vi "单个流程写入.vi"(8 "error in (no error)":errorcluster, 10 "添加的路径":path, 11 "参数簇":T1={"启动参数"=1, "启动模式"=enum."跨度核查", "量程"=enum."低量程"} {"启动参数" items=["总磷"=1, "总氮"=2, "氨氮"=3]}) -> (0 "error out":errorcluster, 3 "步数":i32)   [LabVIEW 2016, in "斯坦道氨氮V2.lvlib"]
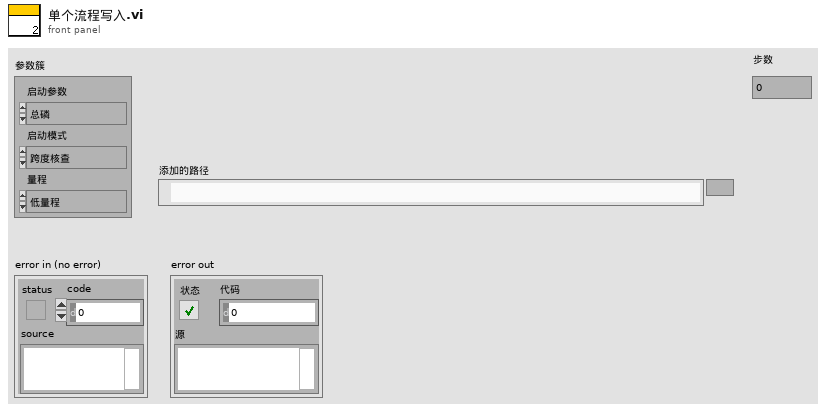
[diagram p1: front panel]
types:
  T1 = cluster{"启动参数":u16, "启动模式":enum16{"跨度核查", "水样测量", "零点核查", "标样核查", "加标回收", "快捷测试", "空白校准", "标样校准"}, "量程":enum16{"低量程", "高量程"}}
  T2 = enum16{"跨度核查", "水样测量", "零点核查", "标样核查", "加标回收", "快捷测试", "空白校准", "标样校准"}
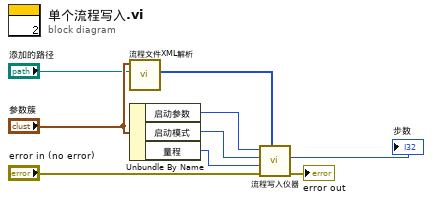
[diagram p0: block diagram]
diagram:
  n1 = call "流程文件XML解析.vi"("添加的路径"="添加的路径", "参数簇"="参数簇") -> ("通讯数据"=w9:u16[])  [unwired: 8 in, 1 out]
  n2 = Unbundle By Name("参数簇") -> ("启动参数"=w7:u16, "启动模式"=w6:T2, "量程"=w5:enum16{"低量程", "高量程"})
  n3 = call "流程写入仪器.vi"("流程"=w9, "error in (no error)"="error in (no error)", "量程"=w5, "测量模式"=w6, "参数"=w7) -> ("error out"=→"error out":errorcluster, "步数"=→"步数":i32)  [unwired: 4 in, 1 out]
